vi "odor-manifold config to port-odor ring entry (sub-vi).vi"(8 "error in (no error)":errorcluster, 10 "odor-manifold config":T3) -> (0 "error out":errorcluster, 2 "ragged ring entry 2D array":T1)   [LabVIEW 2021]
uses:
  type-defs/odor and manifold config cluster (type def).ctl
  type-defs/manifold configuration cluster array (type def).ctl
  type-defs/manifold configuration cluster (type def).ctl
  type-defs/manifold selection.ctl
  type-defs/single port single odor cluster.ctl
  type-defs/port number (type def).ctl
  type-defs/odor selection (type def).ctl
  type-defs/odor color (type def).ctl
  type-defs/odor description array (type def).ctl
  type-defs/odor info cluster (type def).ctl
  type-defs/ragged ring entry 2D array cluster (typed def).ctl
  type-defs/ring string and value cluster (type def).ctl
  global-variables/global variables.vi
  <vilib>/Utility/error.llb/Error Cluster From Error Code.vi
  <vilib>/ErrorRing/Error Ring.xnode
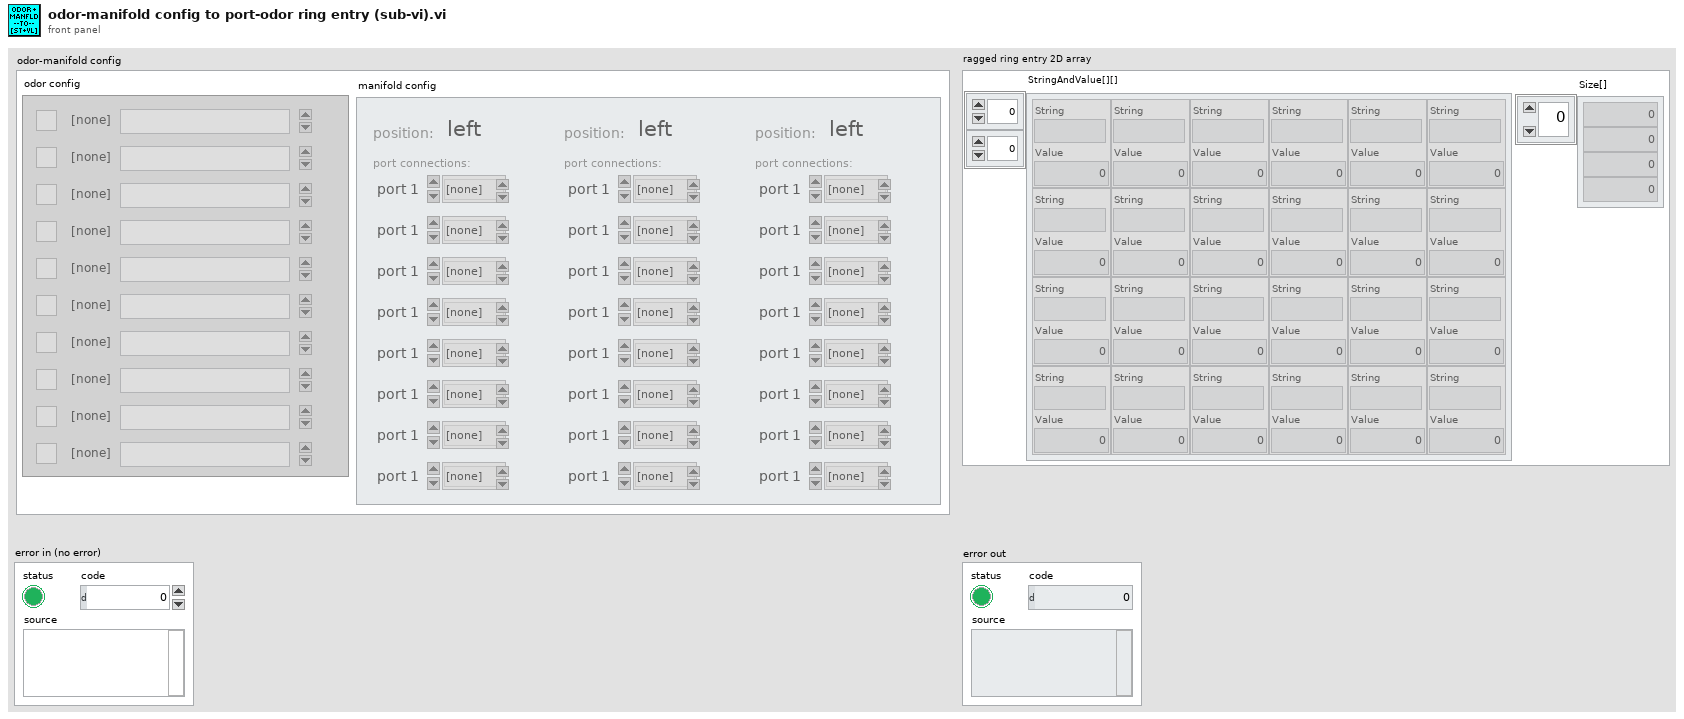
[diagram p1: front panel]
types:
  T1 = typedef "ragged ring entry 2D array cluster (typed def).ctl" = cluster{"StringAndValue[][]":T2[][], "Size[]":i32[]}
  T2 = typedef "ring string and value cluster (type def).ctl" = cluster{"String":string, "Value":u16}
  T3 = typedef "odor and manifold config cluster (type def).ctl" = cluster{"manifold config":T4, "odor config":T11}
  T4 = typedef "manifold configuration cluster array (type def).ctl" = T5[]
  T5 = typedef "manifold configuration cluster (type def).ctl" = cluster{"position:":T6, "port connections:":T7[]}
  T6 = typedef "manifold selection.ctl" = enum16{"left", "middle", "right"}
  T7 = typedef "single port single odor cluster.ctl" = cluster{"port number":T8, "connected odor":T9, "error":bool, "odor color":T10}
  T8 = typedef "port number (type def).ctl" = enum16{"port 1", "port 2", "port 3", "port 4", "port 5", "port 6", "port 7", "port 8"}
  T9 = typedef "odor selection (type def).ctl" = enum16{"[none]", "odor 1", "odor 2", "odor 3", "odor 4", "odor 5", "odor 6", "odor 7", "odor 8", "odor 9", "odor 10"}
  T10 = typedef "odor color (type def).ctl" = u16
  T11 = typedef "odor description array (type def).ctl" = T12[]
  T12 = typedef "odor info cluster (type def).ctl" = cluster{"odor channel":T9, "odor description":string, "odor color":T10, "odor channel active":bool}
  T13 = typedef "odor channel to string map (type def).ctl" = map{T9, string}
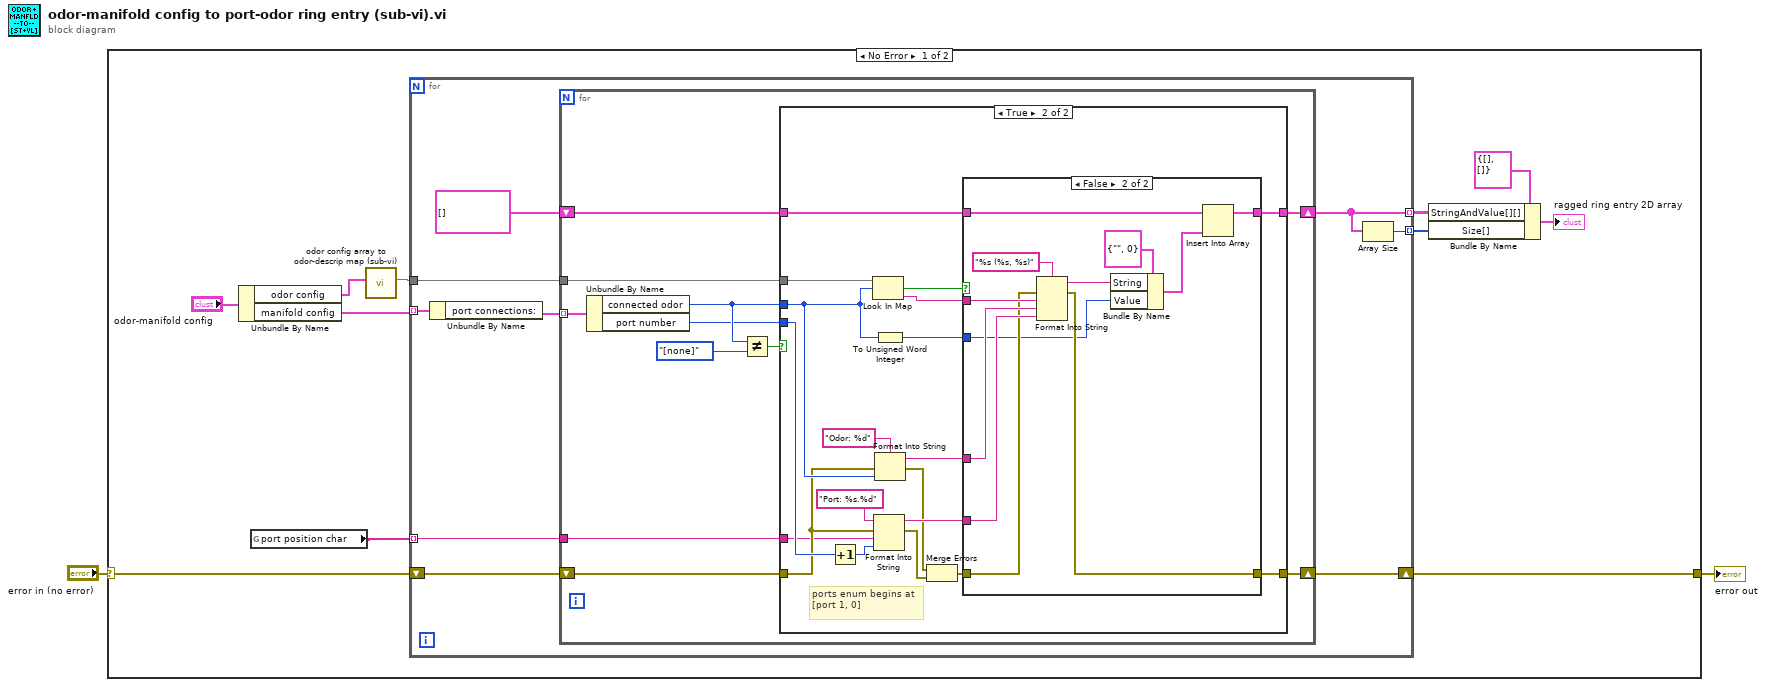
[diagram p0: block diagram]
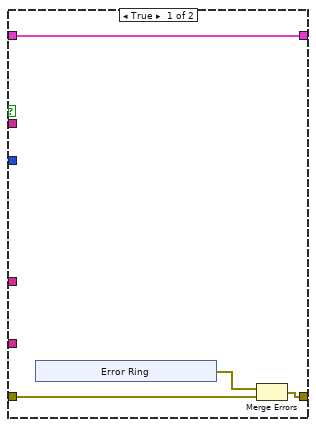
[diagram p3: hidden frame]
diagram:
  n1 = case shown="No Error" "error in (no error)" {
    selector: "error in (no error)" -> [w5 w76]
    tunnel: [w4 w76] -> w1
    frame No Error {
      n2 = Unbundle By Name("odor-manifold config") -> ("odor config"=w10:T11, "manifold config"=w11:T4)
      n3 = global read "global variables.vi" "port position char"() -> (w3:string[])
      n4 = call "odor config array to odor-descrip map (sub-vi).vi"("odor config array"=w10) -> ("odor channel to description map"=w12:T13)  [unwired: 10 in]
      n5 = for {
        tunnel: w11 -> [w21] mode=indexing
        tunnel: w12 -> [w20]
        tunnel: [w18] -> w7 mode=indexing
        tunnel: [w17] -> w8 mode=indexing
        shift-right: [w15] -> w4
        shift-left: w5 -> [w16]
        tunnel: w3 -> [w14] mode=indexing
        n6 = Unbundle By Name(w21) -> ("port connections:"=w22:T7[])
        n7 = for {
          tunnel: w22 -> [w33] mode=indexing
          shift-right: [w32] -> w18
          shift-left: T2[] [] -> [w31]
          tunnel: w20 -> [w28]
          shift-right: [w25] -> w15
          shift-left: w16 -> [w24]
          tunnel: w14 -> [w23]
          n8 = Unbundle By Name(w33) -> ("connected odor"=w27:T9, "port number"=w26:T8)
          n9 = Not Equal?(x=w27, y=odor_selection_(type_def)."[none]" ("connected odor")) -> (x != y?=w29:bool)
          n10 = case shown="True" w29 {
            tunnel: [w35 w48] -> w32
            tunnel: w31 -> [w35 w54]
            tunnel: w27 -> [_ w46]
            tunnel: w28 -> [_ w51]
            tunnel: w26 -> [_ w47]
            tunnel: [w34 w39] -> w25
            tunnel: w24 -> [w34 w38]
            tunnel: w23 -> [_ w36]
            frame False {
            }
            frame True {
              # "ports enum begins at \n[port 1, 0]"
              n11 = Increment(x=w47) -> (x+1=w37:T8)
              n12 = Look In Map(map=w51, key=w46) -> (key not found?=w50:bool, value=w49:string)  [unwired: 1 in]
              n13 = Format Into String(format string="Port: %s.%d", error in=w38, w36, w37) -> (resulting string=w44:string, error out=w42:errorcluster)  [unwired: 1 in]
              n14 = To Unsigned Word Integer(number=w46) -> (unsigned 16bit integer=w40:u16)
              n15 = Format Into String(format string="Odor: %d", error in=w38, w46) -> (resulting string=w45:string, error out=w43:errorcluster)  [unwired: 1 in]
              n16 = Merge Errors(w43, w42) -> (w41:errorcluster)
              n17 = case shown="False" w50 {
                tunnel: w54 -> [w58 w75]
                tunnel: w49 -> [_ w73]
                tunnel: w45 -> [_ w72]
                tunnel: w44 -> [_ w71]
                tunnel: [w58 w70] -> w48
                tunnel: w41 -> [w57 w65]
                tunnel: [w55 w66] -> w39
                tunnel: w40 -> [_ w64]
                frame True {
                  n18 = xnode "Error Ring"() -> ("error out"=w56:errorcluster)
                  n19 = Merge Errors(w56, w57) -> (w55:errorcluster)
                }
                frame False {
                  n20 = Format Into String(format string="%s (%s, %s)", error in=w65, w73, w72, w71) -> (resulting string=w68:string, error out=w66:errorcluster)  [unwired: 1 in]
                  n21 = Bundle By Name(cluster=T2 {"String"="", "Value"=0} ("output cluster"), "String"=w68, "Value"=w64) -> (w67:T2)
                  n22 = Insert Into Array(array=w75, new element=w67) -> (w70:T2[])  [unwired: 1 in]
                }
              }
            }
          }
        }
        n23 = Array Size(array=w18) -> (size(s)=w17:i32)
      }
      n24 = Bundle By Name(cluster=T1 {"StringAndValue[][]"=[], "Size[]"=[]} ("ragged ring entry 2D array"), "StringAndValue[][]"=w7, "Size[]"=w8) -> (→"ragged ring entry 2D array":T1)
    }
    frame Error {
    }
  }
  "error out" <- w1
